vi "Update Template Plugin Files.vi"(8 "error in":errorcluster, 10 "plugin library path":path, 11 "configuration":T1) -> (0 "error out":errorcluster)   [LabVIEW 2021, in "InstrumentStudio Plug-In Editor.lvlib"]
uses:
  InstrumentStudio Plug-In Editor.lvlib
  Data Holder.ctl
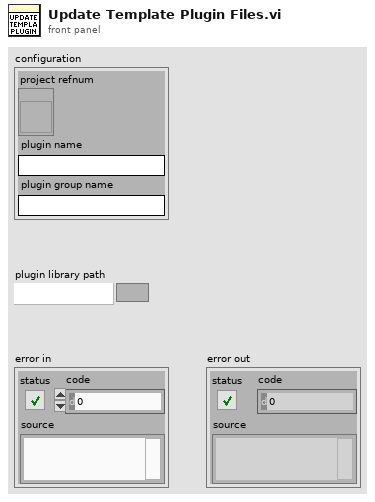
[diagram p1: front panel]
types:
  T1 = typedef "InstrumentStudio Plug-In Editor.lvlib/Data Holder.ctl" = cluster{"project refnum":refnum<vi>, "plugin name":string, "plugin group name":string}
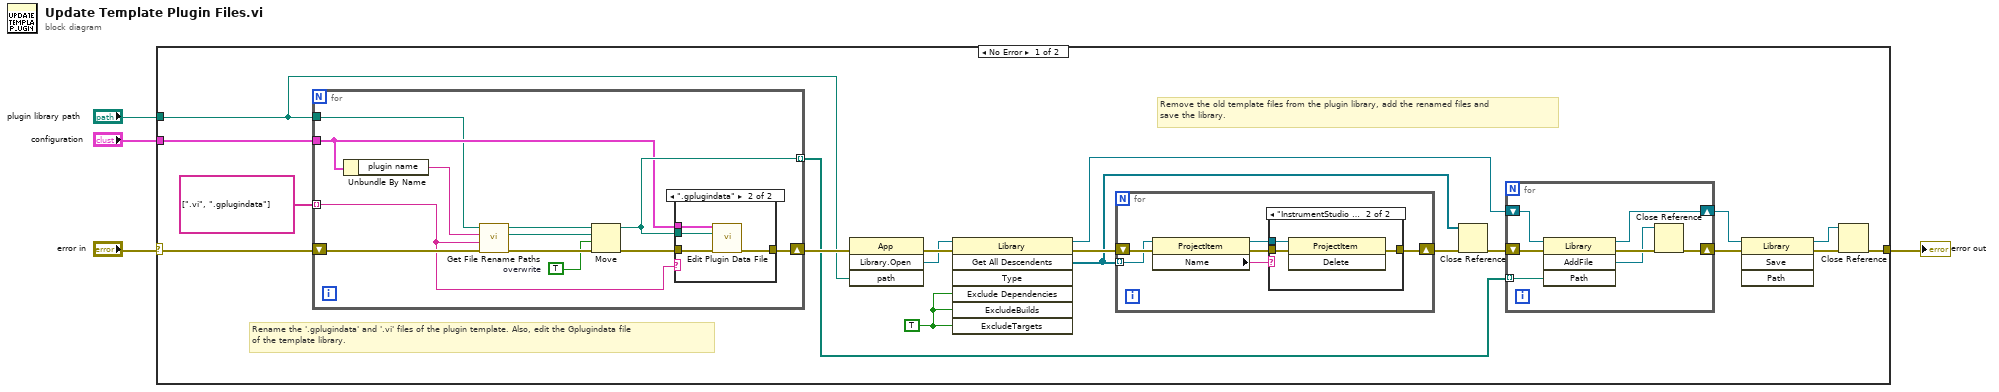
[diagram p0: block diagram]
diagram:
  n1 = case shown="No Error" "error in" {
    selector: "error in" -> [w23 w58]
    tunnel: [w9 w58] -> w4
    tunnel: "configuration" -> [w8 _]
    tunnel: "plugin library path" -> [w7 _]
    frame No Error {
      w6 = TRUE ("ExcludeDependencies")
      # "Remove the old template files from the plugin library, add the renamed files and\nsave the library."
      # "Rename the '.gplugindata' and '.vi' files of the plugin template. Also, edit the Gplugindata file\nof the template library."
      n2 = for {
        shift-right: [w34] -> w11
        shift-left: w23 -> [w33]
        tunnel: [w28] -> w10 mode=indexing
        tunnel: w8 -> [w27]
        tunnel: w7 -> [w26]
        tunnel: string[] [".vi", ".gplugindata"] -> [w24] mode=indexing
        w25 = TRUE  # overwrite
        n3 = Unbundle By Name(w27) -> ("plugin name"=w29:string)
        n4 = call "Get File Rename Paths.vi"("error in"=w33, "plugin file format"=w24, "plugin name"=w29, "plugin library path"=w26) -> ("error out"=w32:errorcluster, "new file path"=w30:path, "old file path"=w31:path)  [unwired: 5 in]
        n5 = Move(source path=w31, error in=w32, 9:w25, 10:w30) -> (error out=w35:errorcluster, 3:w28:path)  [unwired: 1 in, 1 out]
        n6 = case shown="\".gplugindata\"" w24 {
          tunnel: w35 -> [w36 w40]
          tunnel: [w36 w39] -> w34
          tunnel: w27 -> [_ w38]
          tunnel: w28 -> [_ w37]
          frame Default {
          }
          frame ".gplugindata" {
            n7 = call "Edit Plugin Data File.vi"("configuration"=w38, "plugin data file path"=w37, "error in"=w40) -> ("error out"=w39:errorcluster)  [unwired: 12 in]
          }
        }
      }
      n8 = invoke class="App" method="Library.Open"(error in=w11, "path"=w7) -> (error out=w22:errorcluster, "Open Library"=w19:refnum<vi>)  [unwired: 2 in, 2 out]
      n9 = invoke class="Library" method="Get All Descendents"(reference=w19, error in=w22, "Exclude Dependencies"=w6, "ExcludeBuilds"=w6, "ExcludeTargets"=w6) -> (reference out=w16:refnum<vi>, error out=w20:errorcluster, "All Descendents"=w12:refnum<vi>[])  [unwired: 2 in, 4 out]
      n10 = for {
        shift-right: [w52] -> w21
        shift-left: w20 -> [w53]
        tunnel: w12 -> [w50] mode=indexing
        n11 = property class="ProjectItem"(reference=w50, error in=w53) -> (reference out=w49:refnum<vi>, error out=w51:errorcluster, "Name"=w48:string)
        n12 = case shown="\"InstrumentStudio Plug-In Template.gplugindata\", \"InstrumentStudio Plug-In Template.vi\"" w48 {
          tunnel: w51 -> [w54 w57]
          tunnel: [w54 w56] -> w52
          tunnel: w49 -> [_ w55]
          frame Default {
          }
          frame "InstrumentStudio Plug-In Template.gplugindata", "InstrumentStudio Plug-In Template.vi" {
            n13 = invoke class="ProjectItem" method="Delete"(reference=w55, error in=w57) -> (error out=w56:errorcluster)  [unwired: 1 in, 2 out]
          }
        }
      }
      n14 = Close Reference(reference=w12, error in (no error)=w21) -> (error out=w18:errorcluster)
      n15 = for {
        shift-right: [w45] -> w17
        shift-left: w18 -> [w47]
        shift-right: [w43] -> w14
        shift-left: w16 -> [w44]
        tunnel: w10 -> [w41] mode=indexing
        n16 = invoke class="Library" method="AddFile"(reference=w44, error in=w47, "Path"=w41) -> (reference out=w43:refnum<vi>, error out=w46:errorcluster, "AddFile"=w42:refnum<vi>)  [unwired: 1 in, 1 out]
        n17 = Close Reference(reference=w42, error in (no error)=w46) -> (error out=w45:errorcluster)
      }
      n18 = invoke class="Library" method="Save"(reference=w14, error in=w17) -> (reference out=w13:refnum<vi>, error out=w15:errorcluster)  [unwired: 2 in, 2 out]
      n19 = Close Reference(reference=w13, error in (no error)=w15) -> (error out=w9:errorcluster)
    }
    frame Error {
    }
  }
  "error out" <- w4
